vi "general plotter variable display info to tcp subsc info.vi"(11 "Array":string[][](array[string])) -> (3 "TCP subscriptions info":T1)   [LabVIEW 2020]
uses:
  Shared/GUI_Template/TCP subscription info cluster.ctl
  <userlib>/_OpenG.lib/array/array.llb/Search 1D Array (String)__ogtk.vi
  <userlib>/_OpenG.lib/array/array.llb/Delete Elements from 2D Array (String)__ogtk.vi
  <userlib>/_OpenG.lib/array/array.llb/Index 1D Array Elements (String)__ogtk.vi
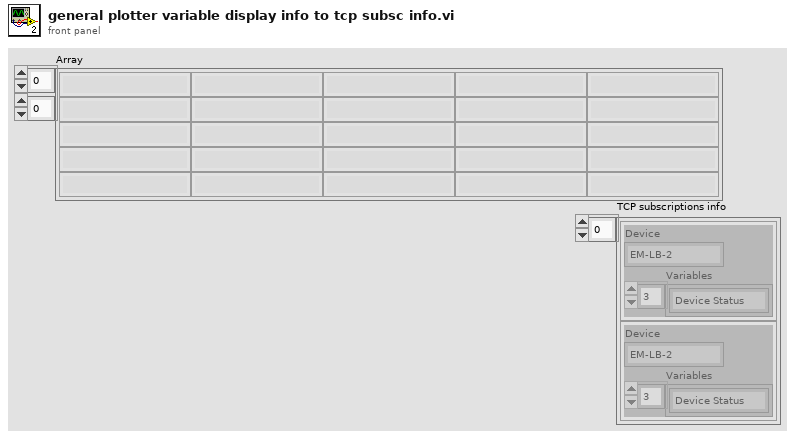
[diagram p1: front panel]
types:
  T1 = typedef "TCP subscription info cluster.ctl" = cluster{"Device":string, "Variables":string[]}[]
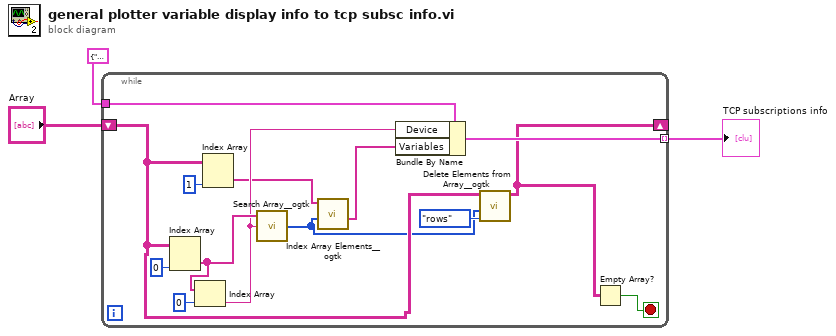
[diagram p0: block diagram]
diagram:
  n1 = while {
    tunnel: cluster{"Device":string, "Variables":string[]} {"Device"="EM-LB-2", "Variables"=["Reading.Channel 1"]} ("Single TCP subscription info") -> [w17]
    tunnel: [w16] -> w2 mode=indexing
    shift-right: [w4] -> _
    shift-left: "Array" -> [w8]
    stop <- w5 stop-if-true
    n2 = Index Array(array=w8, index (col)=0 ("disabled index (col)")) -> (element=w14:string[])  [unwired: 1 in]
    n3 = Index Array(array=w14, index=0) -> (element=w12:string)
    n4 = Index Array(array=w8, index (col)=1 ("disabled index (col)")) -> (element=w10:string[])  [unwired: 1 in]
    n5 = call-poly <userlib>:"Search Array__ogtk.vi"("Array"=w14, "Element Data"=w12) -> ("Indices of Elements"=w6:i32[])  [unwired: 7 in]
    n6 = call-poly <userlib>:"Index Array Elements__ogtk.vi"("indices"=w6, "array"=w10) -> ("elements"=w9:string[])  [unwired: 9 in]
    n7 = Bundle By Name(cluster=w17, "Device"=w12, "Variables"=w9) -> (w16:cluster{"Device":string, "Variables":string[]})
    n8 = call-poly <userlib>:"Delete Elements from Array__ogtk.vi"("delete (rows or columns)"=enum16{"rows", "columns"}."rows", "indices"=w6, "array"=w8) -> ("array w/ subset deleted"=w4:string[][])  [unwired: 7 in, 1 out]
    n9 = Empty Array?(array=w4) -> (empty?=w5:bool)
  }
  "TCP subscriptions info" <- w2
